vi "calc_text_width.vi"(10 "String":string, 11 "Scene Text Object":refnum<vi>) -> (2 "Estimated Text Width":dbl min=-1.7976931348623157e+308 max=1.7976931348623157e+308, 3 "Scene Text Out":refnum<vi>)   [LabVIEW 2020, in "3DPC_SurfacePlot.xctl"]
uses:
  <vilib>/Native 3D Graph/xcontrol/3DPC_SurfacePlot.xctl
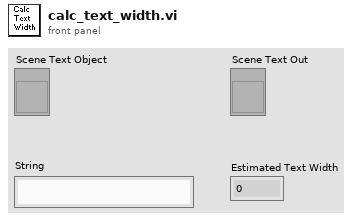
[diagram p1: front panel]
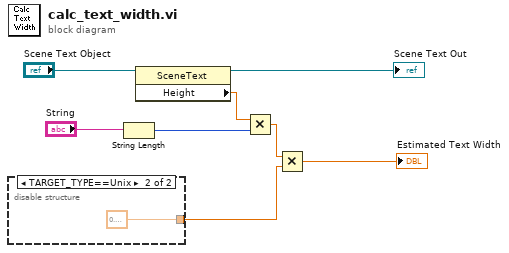
[diagram p0: block diagram]
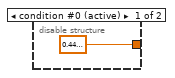
[diagram p2: hidden frame]
diagram:
  n1 = disable-structure shown="TARGET_TYPE==Unix" {
    disable-tunnel: [sgl 0.45 ("y") sgl 0.8 ("y")] -> w1
    frame condition #0 (active) {
    }
    frame condition #1 {
    }
  }
  n2 = String Length(string="String") -> (length=w5:i32)
  n3 = property class="SceneText"(reference="Scene Text Object") -> (reference out=→"Scene Text Out":refnum<vi>, "Height"=w6:sgl)  [unwired: 1 in, 1 out]
  n4 = Multiply(x=w6, y=w5) -> (x*y=w3:sgl)
  n5 = Multiply(x=w3, y=w1) -> (x*y=→"Estimated Text Width":sgl)
